vi "VIQA Password.vi"(8 "error in (no error)":errorcluster, 9 "Skip All? (F)":bool, 11 "VI Refnum":refnum<vi>) -> (0 "error out":errorcluster, 1 "Skip All?":bool, 2 "Locked":bool, 3 "dup VI Refnum":refnum<vi>)   [LabVIEW 2018, in "VI Quality.lvlib"]
uses:
  VI Quality.lvlib
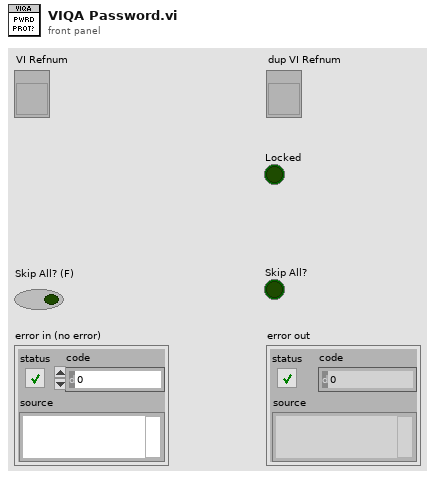
[diagram p1: front panel]
types:
  T1 = enum32{"invalid lock state", "Not Locked", "Locked (No Password)", "Password-protected"}
  T2 = enum16{"Left Button", "Center Button", "Right Button", "Window Close"}
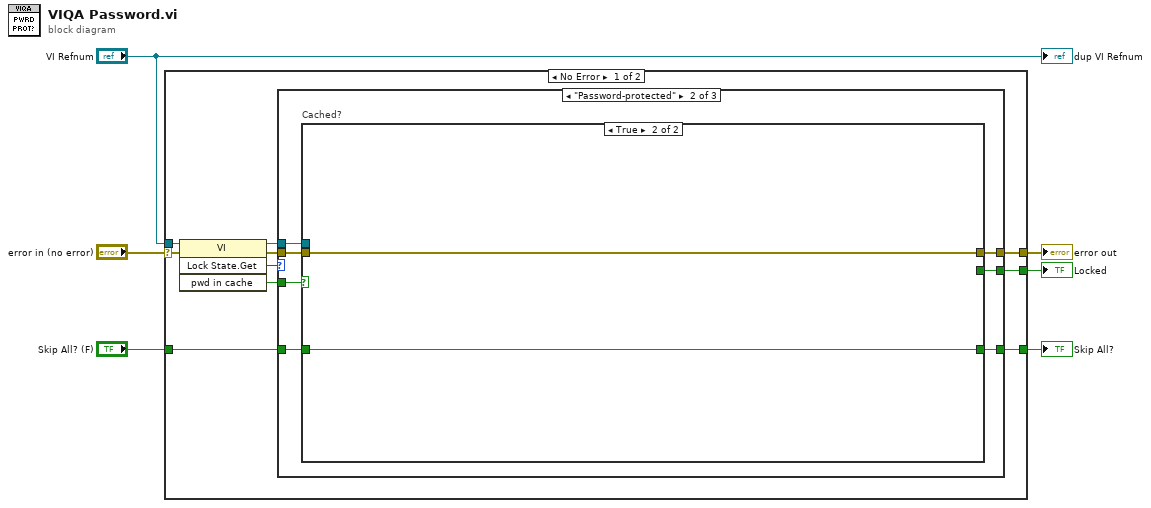
[diagram p0: block diagram]
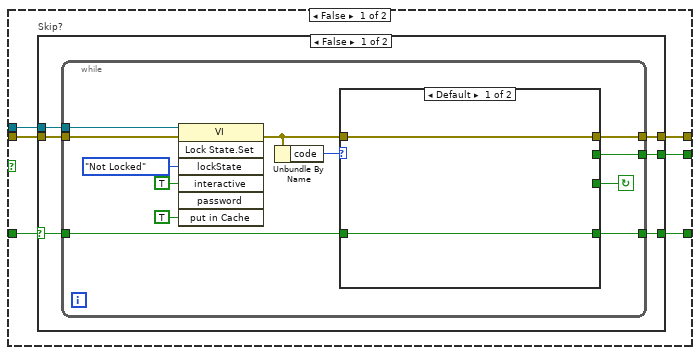
[diagram p3: hidden frame]
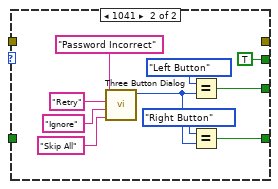
[diagram p4: hidden frame]
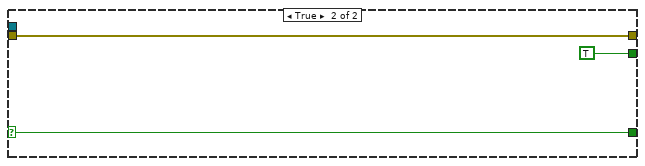
[diagram p5: hidden frame]
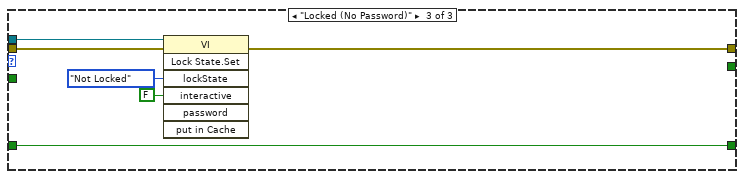
[diagram p6: hidden frame]
diagram:
  n1 = case shown="No Error" "error in (no error)" {
    selector: "error in (no error)" -> [w15 w74]
    tunnel: "VI Refnum" -> [w16 _]
    tunnel: [w10 _] -> w4
    tunnel: [w12 w74] -> w3
    tunnel: "Skip All? (F)" -> [w11 w73]
    tunnel: [w8 w73] -> w1
    frame No Error {
      n2 = invoke class="VI" method="Lock State.Get"(reference=w16, error in=w15) -> (reference out=w13:refnum<vi>, error out=w14:errorcluster, "Get Lock State"=w9:T1, "pwd in cache"=w7:bool)  [unwired: 2 in]
      n3 = case shown="\"Password-protected\"" w9 {
        tunnel: w14 -> [w18 w25 w69]
        tunnel: w13 -> [_ w24 w70]
        tunnel: [w18 w23 w68] -> w12
        tunnel: w11 -> [w17 w22 w67]
        tunnel: [_ w21 _] -> w10
        tunnel: [w17 w20 w67] -> w8
        tunnel: w7 -> [_ w19 _]
        frame Default {
        }
        frame "Password-protected" {
          n4 = case "Cached?" shown="True" w19 {
            tunnel: w25 -> [w31 w66]
            tunnel: w24 -> [w30 _]
            tunnel: [w29 w66] -> w23
            tunnel: w22 -> [w28 w65]
            tunnel: [w27 _] -> w21
            tunnel: [w26 w65] -> w20
            frame False {
              n5 = case "Skip?" shown="False" w28 {
                selector: w28 -> [w32 w62]
                tunnel: w31 -> [w37 w64]
                tunnel: w30 -> [w36 _]
                tunnel: [w35 w64] -> w29
                tunnel: [w33 TRUE] -> w27
                tunnel: [w34 w62] -> w26
                frame False {
                  n6 = while {
                    tunnel: w37 -> [w49]
                    tunnel: w36 -> [w48]
                    tunnel: [w42] -> w35
                    tunnel: [w41] -> w34
                    tunnel: [w39] -> w33
                    tunnel: w32 -> [w38]
                    stop <- w40 continue-if-true
                    n7 = invoke class="VI" method="Lock State.Set"(reference=w48, error in=w49, "lockState"=T1."Not Locked" ("Lock State"), "interactive"=TRUE ("Interactive"), "put in Cache"=TRUE ("Put in Cache")) -> (error out=w43:errorcluster)  [unwired: 2 in, 6 out]
                    n8 = Unbundle By Name(w43) -> ("code"=w44:i32)
                    n9 = case shown="Default" w44 {
                      tunnel: w43 -> [w51 _]
                      tunnel: [w51 _] -> w42
                      tunnel: [_ w56] -> w40
                      tunnel: [w50 w53] -> w41
                      tunnel: [_ TRUE] -> w39
                      tunnel: w38 -> [w50 _]
                      frame Default {
                      }
                      frame 1041 {
                        n10 = call <vilib>:"Three Button Dialog.vi"("Right Button Text (\"Cancel\")"="Skip All" ("T button name (\"OK\")"), "Center Button Text (\"No\")"="Ignore" ("T button name (\"OK\")"), "Left Button Text (\"Yes\")"="Retry" ("T button name (\"OK\")"), "message"="Password Incorrect") -> ("Which Button?"=w54:T2)  [unwired: 7 in]
                        n11 = Equal?(x=T2."Left Button" ("y"), y=w54) -> (x = y?=w56:bool)
                        n12 = Equal?(x=T2."Right Button" ("y"), y=w54) -> (x = y?=w53:bool)
                      }
                    }
                  }
                }
                frame True {
                }
              }
            }
            frame True {
            }
          }
        }
        frame "Locked (No Password)" {
          n13 = invoke class="VI" method="Lock State.Set"(reference=w70, error in=w69, "lockState"=T1."Not Locked" ("Lock State"), "interactive"=FALSE ("Interactive")) -> (error out=w68:errorcluster)  [unwired: 3 in, 6 out]
        }
      }
    }
    frame Error {
    }
  }
  "error out" <- w3
  "Locked" <- w4
  "Skip All?" <- w1
  "dup VI Refnum" <- "VI Refnum"
